vi "Operaciones_Senales_3.vi"() -> ()   [LabVIEW 2016]
uses:
  <vilib>/DAQmx/read.llb/DAQmx Read (Analog 1D DBL 1Chan NSamp).vi
  <vilib>/DAQmx/write.llb/DAQmx Write (Analog 2D DBL NChan NSamp).vi
  <vilib>/DAQmx/create/channels.llb/DAQmx Create Channel (AI-Voltage-Basic).vi
  <vilib>/DAQmx/configure/timing.llb/DAQmx Timing (Sample Clock).vi
  <vilib>/DAQmx/miscellaneous.llb/DAQmx Fill In Error Info.vi
  <vilib>/DAQmx/create/channels.llb/DAQmx Create Channel (AO-Voltage-Basic).vi
  <vilib>/imath/engines/lvmath2/RunTimeEngine/BuiltInFunctions/length/NIMS_length(GV).vi
  <instcachedir>/0/NIMS_length(GV)_08A3D13377FD4E4B96F5795FBF3698FA.lvgen/NIMS_length(GV)_08A3D13377FD4E4B96F5795FBF3698FA_000.vi
  <vilib>/imath/engines/lvmath2/RunTimeEngine/RangeToken/NIMS_Range.vi
  <instcachedir>/0/NIMS_Range_A7C094595B484CA7AF10685B02D808ED.lvgen/NIMS_Range_A7C094595B484CA7AF10685B02D808ED_001.vi
  <vilib>/imathl/engines/lvmath/Functions/Error Handling/Create Error.vi
  <vilib>/imath/engines/lvmath2/RunTimeEngine/IndexReplace/NIMS V(S)=S.vi
  <instcachedir>/0/NIMS V(S)=S_57E16554CB8B4B90AAB163894F717546.lvgen/NIMS V(S)=S_57E16554CB8B4B90AAB163894F717546_003.vi
  <vilib>/imath/engines/lvmath2/RunTimeEngine/RangeToken/NIMS_Range_R2 - Integer.vi
  <instcachedir>/0/NIMS_Range_R2 - Integer_89B873E74E6E489885E44F751DD9C6BF.lvgen/NIMS_Range_R2 - Integer_89B873E74E6E489885E44F751DD9C6BF_000.vi
  <vilib>/imath/engines/lvmath2/RunTimeEngine/CommandStatement/MC_CommandStatement_break.vi
  <vilib>/imath/engines/lvmath2/RunTimeEngine/IndexRead/NIMS V(S).vi
  <instcachedir>/0/NIMS V(S)_0488751826AF41519A22953C041130DC.lvgen/NIMS V(S)_0488751826AF41519A22953C041130DC_000.vi
  <instcachedir>/0/NIMS V(S)=S_57E16554CB8B4B90AAB163894F717546.lvgen/NIMS V(S)=S_57E16554CB8B4B90AAB163894F717546_000.vi
  <vilib>/imath/engines/lvmath2/RunTimeEngine/ErrorHandling/NIMS_Create Error From Enums.vi
  <vilib>/imath/engines/lvmath2/RunTimeEngine/NodeEndStatement/NIMS_NodeEndStatement_Output.vi
  <instcachedir>/0/NIMS_NodeEndStatement_Output_53EC0D466D134D7ABD903AC30B43404B.lvgen/NIMS_NodeEndStatement_Output_53EC0D466D134D7ABD903AC30B43404B_005.vi
  <vilib>/imath/engines/lvmath2/RunTimeEngine/ErrorHandling/NIMS_Finalize Error.vi
  <vilib>/Waveform/WDTFileIO.llb/ Write Waveform to File.vi
panel:
  in  "file path (dialog if empty) 2":path
  in  "file path (dialog if empty)":path
  out "Integral":cluster{"Tiempo":dbl[], "Entrada":dbl[]}(graph)
  out "Derivada":cluster{"Tiempo":dbl[], "Entrada":dbl[]}(graph)
  out "Entrada":cluster{"Tiempo":dbl[], "Entrada":dbl[]}(graph)
  out "data":dbl[](graph)
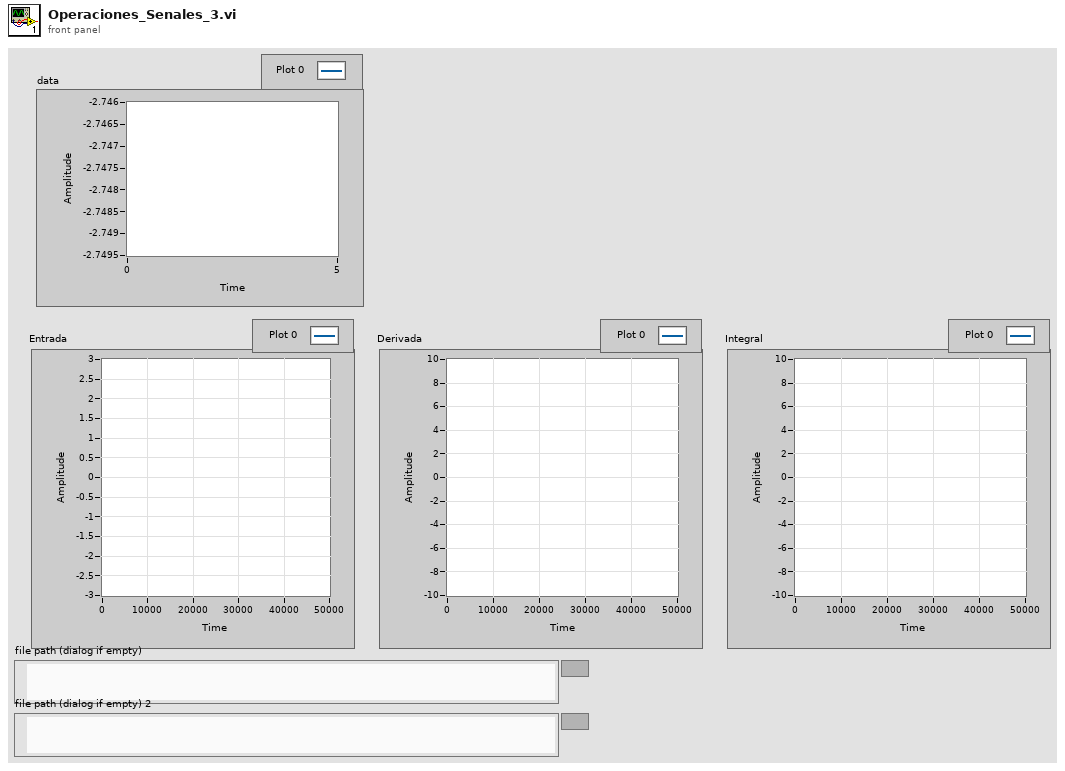
[diagram p1: front panel]
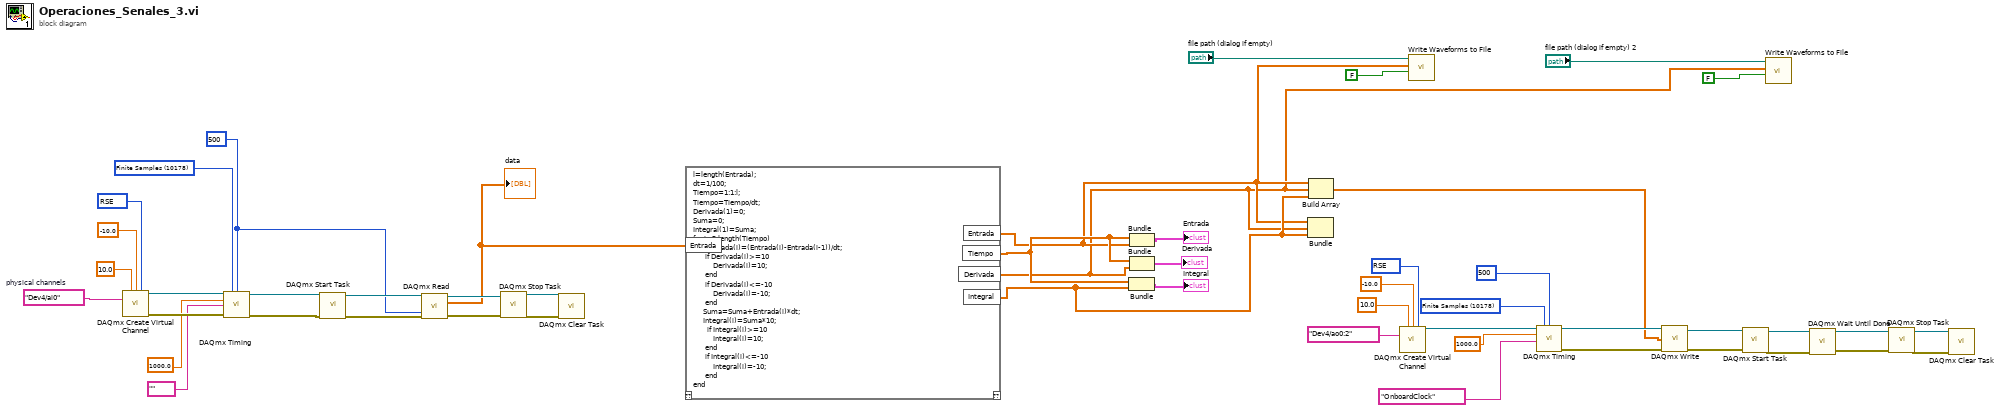
[diagram p0: block diagram]
diagram:
  w23 = 10178 items=["Finite Samples"=10178, "Continuous Samples"=10123, "Hardware Timed Single Point"=12522] ("sample mode")
  w28 = 10083 items=["Default"=-1, "RSE"=10083, "Differential"=10106, "Pseudodifferential"=12529] ("output terminal configuration")
  w37 = 500 ("samples per channel")
  w46 = 10178 items=["Finite Samples"=10178, "Continuous Samples"=10123, "Hardware Timed Single Point"=12522] ("sample mode")
  w47 = tag "Dev4/ai0"  # physical channels
  w50 = 10083 items=["Default"=-1, "RSE"=10083, "NRSE"=10078, "Differential"=10106, "Pseudodifferential"=12529] ("input terminal configuration")
  n1 = call-poly <vilib>:"DAQmx Create Virtual Channel.vi"("maximum value"=10.0, "minimum value"=-10.0, "input terminal configuration"=w50, "physical channels"=w47) -> ("task out"=w45:refnum<k21>, "error out"=w44:errorcluster)  [unwired: 10 in]
  n2 = call-poly <vilib>:"DAQmx Timing.vi"("task/channels in"=w45, "sample mode"=w46, "samples per channel"=w37, "rate"=1000.0, "source"=tag "", "error in"=w44) -> ("task out"=w41:refnum<k21>, "error out"=w39:errorcluster)  [unwired: 8 in]
  n3 = call <vilib>:"DAQmx Start Task.vi"("task/channels in"=w41, "error in"=w39) -> ("task out"=w40:refnum<k21>, "error out"=w38:errorcluster)  [unwired: 12 in]
  n4 = call-poly <vilib>:"DAQmx Read.vi"("task/channels in"=w40, "timeout"=w37, "error in"=w38) -> ("task out"=w35:refnum<k21>, "data"=w32:dbl[], "error out"=w36:errorcluster)  [unwired: 10 in]
  "data" <- w32
  n5 = call <vilib>:"DAQmx Stop Task.vi"("task/channels in"=w35, "error in"=w36) -> ("task out"=w34:refnum<k21>, "error out"=w33:errorcluster)  [unwired: 12 in]
  n6 = call <vilib>:"DAQmx Clear Task.vi"("task in"=w34, "error in"=w33) -> ()  [unwired: 13 in, 1 out]
  n7 = mathscript code="l=length(Entrada);\ndt=1/100;\nTiempo=1:1:l;\nTiempo=Tiempo/dt;\nDerivada(1)=0;\nSuma=0;\nIntegral(1)=Suma;\nfor i=2:length(Tiempo)\n     Derivada(i)=(Entrada(i)-Entrada(i-1))/dt;\n      if Derivada(i)>=10 \n          Derivada(i)=10;\n      end\n      if Derivada(i)<=-10 \n          Derivada(i)=-10;\n      end\n     Suma=Suma+Entrada(i)*dt;\n     Integral(i)=Suma*10;\n       if Integral(i)>=10 \n          Integral(i)=10;\n      end\n      if Integral(i)<=-10 \n          Integral(i)=-10;\n      end\nend"("Entrada"=w32) -> ("Entrada"=w6:dbl[], "Tiempo"=w11:dbl[], "Derivada"=w1:dbl[], "Integral"=w10:dbl[])  [unwired: 1 in, 1 out]
  n8 = Bundle("Tiempo"=w11, "Integral"=w10) -> (→"Integral":cluster{"Tiempo":dbl[], "Integral":dbl[]})  [unwired: 1 in]
  n9 = Bundle("Tiempo"=w11, "Entrada"=w6) -> (→"Entrada":cluster{"Tiempo":dbl[], "Entrada":dbl[]})  [unwired: 1 in]
  n10 = Bundle("Tiempo"=w11, "Derivada"=w1) -> (→"Derivada":cluster{"Tiempo":dbl[], "Derivada":dbl[]})  [unwired: 1 in]
  n11 = Bundle("Entrada"=w6, "Derivada"=w1, "Integral"=w10) -> ()  [unwired: 1 in, 1 out]
  n12 = Build Array(w6, w1, w10) -> (w9:dbl[][])
  n13 = call-poly <vilib>:"DAQmx Create Virtual Channel.vi"("maximum value"=10.0, "minimum value"=-10.0, "output terminal configuration"=w28, "physical channels"=tag "Dev4/ao0:2") -> ("task out"=w25:refnum<k21>)  [unwired: 10 in, 1 out]
  n14 = call-poly <vilib>:"Write Waveforms to File.vi"("append to file? (new file:F)"=FALSE, "waveform"=w6, "file path (dialog if empty)"="file path (dialog if empty)") -> ()  [unwired: 7 in, 2 out]
  n15 = call-poly <vilib>:"DAQmx Timing.vi"("task/channels in"=w25, "sample mode"=w23, "samples per channel"=500, "rate"=1000.0, "source"=tag "OnboardClock") -> ("task out"=w21:refnum<k21>, "error out"=w20:errorcluster)  [unwired: 9 in]
  n16 = call-poly <vilib>:"DAQmx Write.vi"("task/channels in"=w21, "data"=w9, "error in"=w20) -> ("task out"=w15:refnum<k21>, "error out"=w14:errorcluster)  [unwired: 10 in, 1 out]
  n17 = call <vilib>:"DAQmx Start Task.vi"("task/channels in"=w15, "error in"=w14) -> ("task out"=w13:refnum<k21>, "error out"=w12:errorcluster)  [unwired: 12 in]
  n18 = call-poly <vilib>:"Write Waveforms to File.vi"("append to file? (new file:F)"=FALSE, "waveform"=w1, "file path (dialog if empty)"="file path (dialog if empty) 2") -> ()  [unwired: 7 in, 2 out]
  n19 = call <vilib>:"DAQmx Wait Until Done.vi"("task/channels in"=w13, "error in"=w12) -> ("task out"=w19:refnum<k21>, "error out"=w18:errorcluster)  [unwired: 12 in]
  n20 = call <vilib>:"DAQmx Stop Task.vi"("task/channels in"=w19, "error in"=w18) -> ("task out"=w17:refnum<k21>, "error out"=w16:errorcluster)  [unwired: 12 in]
  n21 = call <vilib>:"DAQmx Clear Task.vi"("task in"=w17, "error in"=w16) -> ()  [unwired: 13 in, 1 out]
